vi "test_ort_find_max.vi"() -> ()   [LabVIEW 2016]
uses:
  <vilib>/rvi/DesktopExecutionNode/Execution/niFpgaDEN_Execute.vi
  <vilib>/rvi/DesktopExecutionNode/DesktopExecutionNode.xnode
panel:
  in  "sampleValidDec":i32=3
  out "cycleMax":dbl[](graph)
  in  "cycleLength":i32
  in  "inputNoiseScale":dbl=500.0
  out "outputValidPoints":T1(array[cluster])
  out "output":T2(array[cluster])
  in  "ort.p.methodParams":T3={"ort.p.winSizeP2"=3, "ort.p.syncPoint"=30, "ort.p.useSyncPoint"=FALSE, "ort.p.bypassAvg"=FALSE, "ort.p.searchBounds"={"maxSearchLower"=0, "maxSearchUpper"=5000}}
  out "inEndOfCycle":bool[](array[boolean])
  out "dataIn":dbl[](graph)
  in  "numTicks":i32=600
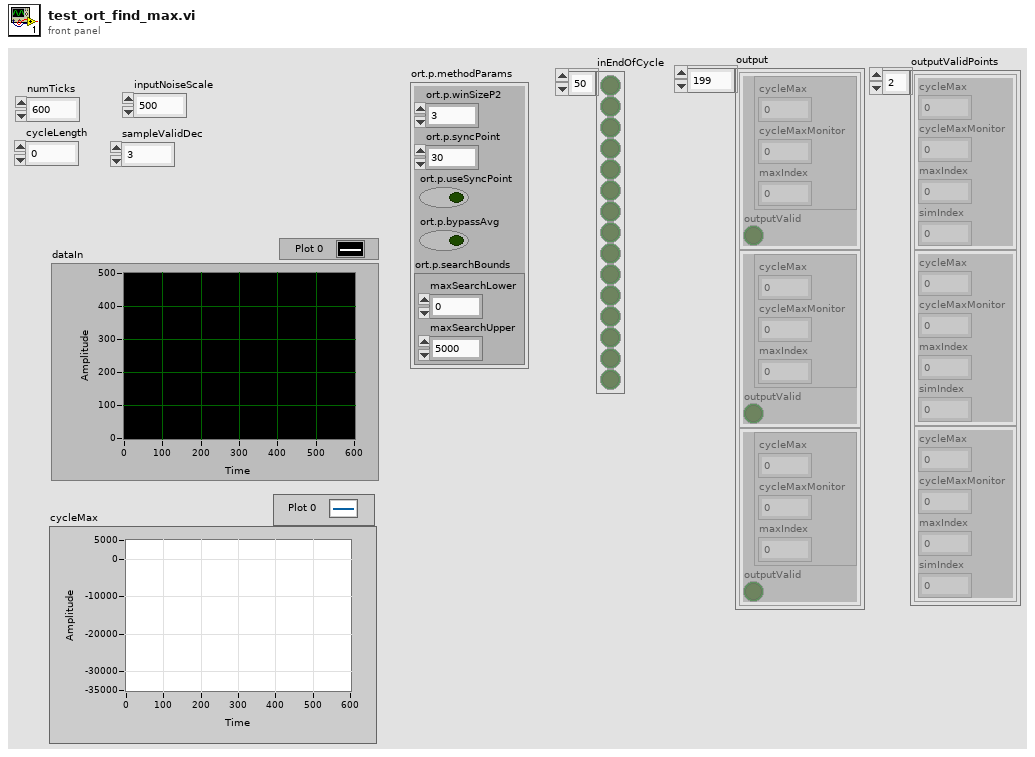
[diagram p1: front panel]
types:
  T1 = cluster{"cycleMax":fxp<+/-,24,16>, "cycleMaxMonitor":fxp<+/-,24,16>, "maxIndex":u16, "simIndex":i32}[]
  T2 = cluster{cluster{"cycleMax":fxp<+/-,24,16>, "cycleMaxMonitor":fxp<+/-,24,16>, "maxIndex":u16}, "outputValid":bool}[]
  T3 = cluster{"ort.p.winSizeP2":u16, "ort.p.syncPoint":u16, "ort.p.useSyncPoint":bool, "ort.p.bypassAvg":bool, "ort.p.searchBounds":cluster{"maxSearchLower":u16, "maxSearchUpper":u16}}
  T4 = cluster{"cycleMax":fxp<+/-,24,16>, "cycleMaxMonitor":fxp<+/-,24,16>, "maxIndex":u16}
  T5 = cluster{cluster{"cycleMax":fxp<+/-,24,16>, "cycleMaxMonitor":fxp<+/-,24,16>, "maxIndex":u16}, "outputValid":bool}
  T6 = cluster{"cycleMax":fxp<+/-,24,16>, "cycleMaxMonitor":fxp<+/-,24,16>, "maxIndex":u16, i32}
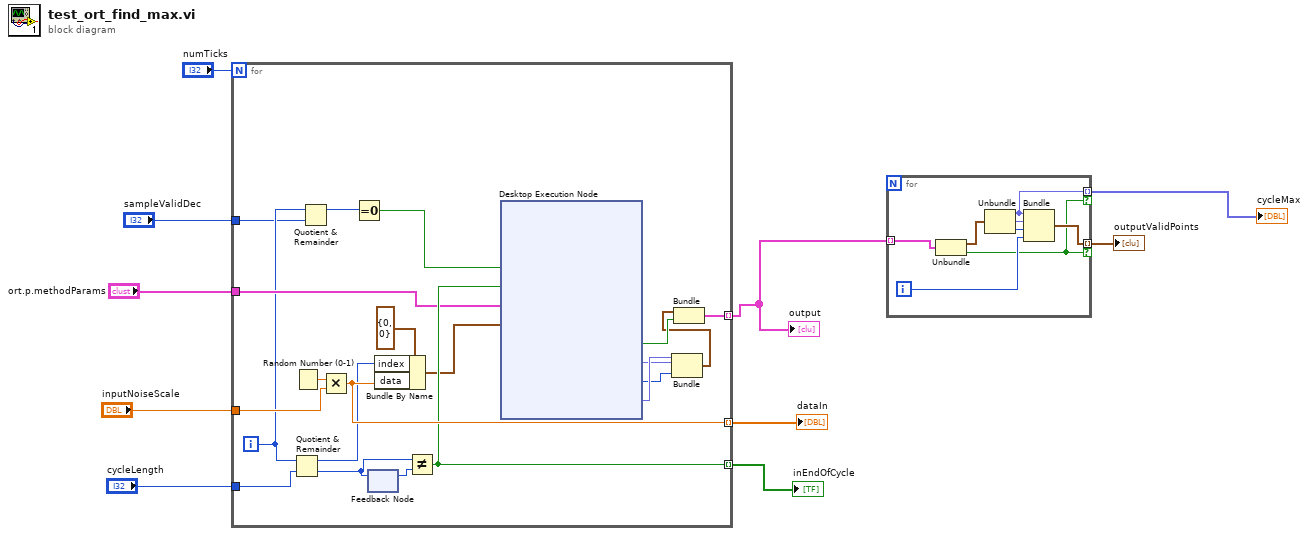
[diagram p0: block diagram]
diagram:
  n1 = for {
    N: "numTicks" -> [_]
    tunnel: [w29] -> w7 mode=indexing
    tunnel: [w28] -> w9 mode=indexing
    tunnel: [w24] -> w8 mode=indexing
    tunnel: "ort.p.methodParams" -> [w23]
    tunnel: "inputNoiseScale" -> [w16]
    tunnel: "cycleLength" -> [w15]
    tunnel: "sampleValidDec" -> [w13]
    i -> [w14]
    n2 = Quotient & Remainder(x=w14, y=w15) -> (x-y*floor(x/y)=w26:i32, floor(x/y)=w25:i32)
    n3 = Random Number (0-1)() -> (number: 0 to 1=w30:dbl)
    n4 = Quotient & Remainder(x=w14, y=w13) -> (x-y*floor(x/y)=w12:i32)  [unwired: 1 out]
    n5 = Multiply(x=w30, y=w16) -> (x*y=w28:dbl)
    n6 = Equal To 0?(x=w12) -> (x = 0?=w11:bool)
    n7 = feedback-in #1(w25) -> ()
    n8 = feedback #1() -> (w27:i32)  [unwired: 1 in]
    n9 = Bundle By Name(cluster=cluster{"index":u16, "data":i16} {"index"=0, "data"=0} ("input"), "index"=w26, "data"=w28) -> (w22:cluster{"index":u16, "data":i16})
    n10 = Not Equal?(x=w25, y=w27) -> (x != y?=w24:bool)
    n11 = xnode "Desktop Execution Node"("inputValid"=w11, "endOfCycle"=w24, "ort.p.methodParams"=w23, "data"=w22) -> ("outputValid"=w21:bool, "cycleMaxMonitor"=w19:fxp<+/-,24,16>, "maxIndex"=w18:u16, "cycleMax"=w20:fxp<+/-,24,16>)  [unwired: 1 in, 1 out]
    n12 = Bundle("cycleMax"=w20, "cycleMaxMonitor"=w19, "maxIndex"=w18) -> (w17:T4)  [unwired: 1 in]
    n13 = Bundle(w17, "outputValid"=w21) -> (w29:T5)  [unwired: 1 in]
  }
  "dataIn" <- w9
  "inEndOfCycle" <- w8
  "output" <- w7
  n14 = for {
    tunnel: w7 -> [w39] mode=indexing
    tunnel: [w36] -> w6 mode=indexing if=w32
    tunnel: [w33] -> w2 mode=indexing if=w32
    i -> [w35]
    n15 = Unbundle(w39) -> (w38:T4, "outputValid"=w32:bool)
    n16 = Unbundle(w38) -> ("cycleMax"=w33:fxp<+/-,24,16>, "cycleMaxMonitor"=w37:fxp<+/-,24,16>, "maxIndex"=w34:u16)
    n17 = Bundle("cycleMax"=w33, "cycleMaxMonitor"=w37, "maxIndex"=w34, w35) -> (w36:T6)  [unwired: 1 in]
  }
  "outputValidPoints" <- w6
  "cycleMax" <- w2
